vi "TrueCounter.vi"(9 "True?":bool) -> (2 "True Count":u16)   [LabVIEW 2018, in "kevLib2010.lvlib"]
doc: "Counts number of trues everytime it is run"
uses:
  kevLib2010.lvlib
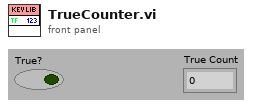
[diagram p1: front panel]
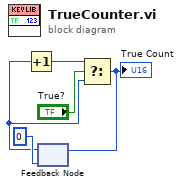
[diagram p0: block diagram]
diagram:
  n1 = feedback #1(u16 0 ("Mismatch Tol")) -> (w3:u16)
  n2 = Increment(x=w3) -> (x+1=w2:u16)
  n3 = Select(t=w2, s="True?", f=w3) -> (s? t:f=w4:u16)
  "True Count" <- w4
  n4 = feedback-in #1(w4) -> ()
